vi "Launcher_SPI.vi"() -> ()   [LabVIEW 2023]
uses:
  SinglePhoton_UI/Libraries/SinglePhotonInterferenceUI/SinglePhotonInterferenceUI/SinglePhotonInterferenceUI.lvclass
  SinglePhoton_UI/Libraries/SPIController/SPIController/SPIController.lvclass
  TranslationStage_UI/TranslationStageUI.lvclass
  <vilib>/ActorFramework/Actor/Actor.lvclass
panel:
  out "Device List":string[][](array[string])
  in  "Control":enum16{"Multiharp", "SPI", "Translation Stages"}(ring)=enum."Translation Stages"
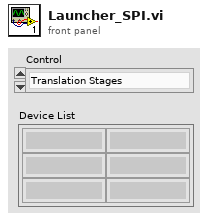
[diagram p1: front panel]
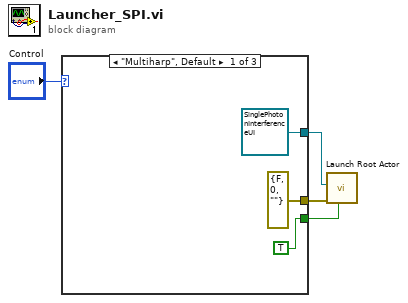
[diagram p0: block diagram]
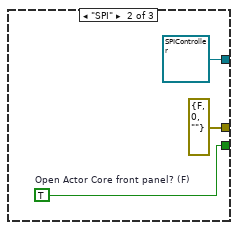
[diagram p2: hidden frame]
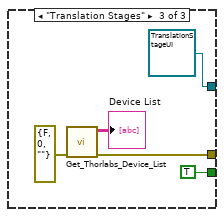
[diagram p3: hidden frame]
diagram:
  n1 = case shown="\"Multiharp\", Default" "Control" {
    tunnel: [TRUE ("Open Actor Core front panel? (F)") w10 TRUE ("Open Actor Core front panel? (F)")] -> w3
    tunnel: [refnum<class "SinglePhotonInterferenceUI.lvclass"> refnum ("SinglePhotonInterferenceUI.lvlib:SinglePhotonInterferenceUI.lvclass") refnum<class "SPIController.lvclass"> refnum ("SPIController.lvlib:SPIController.lvclass") refnum<class "TranslationStageUI.lvclass"> refnum ("TranslationStage_UI.lvlib:TranslationStageUI.lvclass")] -> w2
    tunnel: [errorcluster {"status"=FALSE, "code"=0, "source"=""} ("error out") errorcluster {"status"=FALSE, "code"=0, "source"=""} ("error out") w11] -> w1
    frame "Multiharp", Default {
    }
    frame "SPI" {
      w10 = TRUE  # Open Actor Core front panel? (F)
    }
    frame "Translation Stages" {
      n2 = call "Get_Thorlabs_Device_List.vi"("error in (no error)"=errorcluster {"status"=FALSE, "code"=0, "source"=""}) -> ("error out"=w11:errorcluster, "Device List"=→"Device List":string[][])  [unwired: 9 in]
    }
  }
  n3 = call <vilib>:"Launch Root Actor.vi"("Open Actor Core front panel? (F)"=w3, "error in (no error)"=w1, "Actor"=w2) -> ()  [unwired: 7 in, 2 out]
